vi "RT-Module Id's.vi"(8 "error in":errorcluster, 9 "RT-Module Id":i32[](array[numeric]), 10 "RT-IP":string[](array[string])) -> (0 "error out":errorcluster)   [LabVIEW 2018, in "Host Main.lvlib"]
doc: "This broadcast Event will give the Respective module if for the Respective Realtime Target.\n_____\nCreated using DQMH Event Scripter 7.0.1.1316."
uses:
  Host Main.lvlib
  RT-Module Id's Argument--cluster.ctl
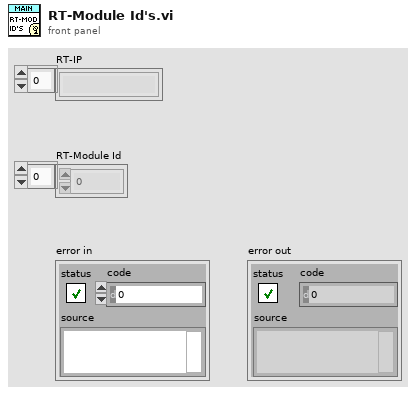
[diagram p1: front panel]
types:
  T1 = typedef "Host Main.lvlib/RT-Module Id's Argument--cluster.ctl" = cluster{"RT-IP":string[], "RT-Module Id":i32[]}
  T2 = typedef "Host Main.lvlib/Broadcast Events--cluster.ctl" = cluster{"Module Did Init":refnum<user-event>, "Status Updated":refnum<user-event>, "Error Reported":refnum<user-event>, "Module Did Stop":refnum<user-event>, "Update Module Execution Status":refnum<user-event>, "RT-Module Id's":refnum<user-event>}
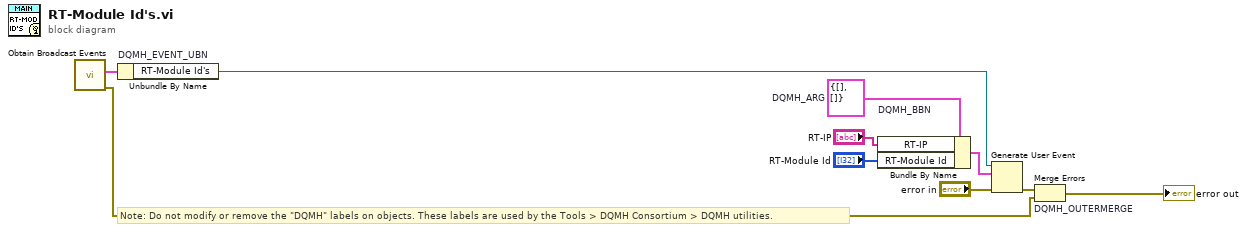
[diagram p0: block diagram]
diagram:
  w5 = T1 {"RT-IP"=[], "RT-Module Id"=[]}  # DQMH_ARG
  # "Note: Do not modify or remove the \"DQMH\" labels on objects. These labels are used by the Tools > DQMH Consortium > DQMH utilities."
  n1 = call "Obtain Broadcast Events.vi"() -> ("error out"=w2:errorcluster, "Host Main Broadcast Events"=w1:T2)  [unwired: 10 in]
  n2 = Unbundle By Name "DQMH_EVENT_UBN"(w1) -> ("RT-Module Id's"=w7:refnum<user-event>)
  n3 = Bundle By Name "DQMH_BBN"(cluster=w5, "RT-IP"="RT-IP", "RT-Module Id"="RT-Module Id") -> (w8:T1)
  n4 = Generate User Event(user event=w7, event data cluster=w8, error in="error in") -> (error out=w6:errorcluster)  [unwired: 1 in, 1 out]
  n5 = Merge Errors "DQMH_OUTERMERGE"(w6, w2) -> (→"error out":errorcluster)
